vi "2_487.vi"() -> ()   [LabVIEW 2018]
uses:
  <vilib>/Utility/config.llb/Write Key (String).vi
  <vilib>/Utility/config.llb/Read Key (String).vi
  <vilib>/Utility/config.llb/NI_LVConfig.lvlib
panel:
  out "字符串":string
  in  "确定按钮 3":bool
  in  "确定按钮 2":bool
  in  "请输入管理密码":string
  out "CANCEL2":bool
  out "OK2":bool
  out "请输入序列号模板2":string
  out "请输入新产品名称2":string
  in  "?":T1
  in  "工号":string
  in  "工序":string
  in  "取消按钮":bool
  in  "确定按钮":bool
  in  "新建":bool
  out "路径":path
  in  "删除":bool
  in  "产品型号":string(combo)
  # "条形码校验系统配置选择"
  # "新建与删除"
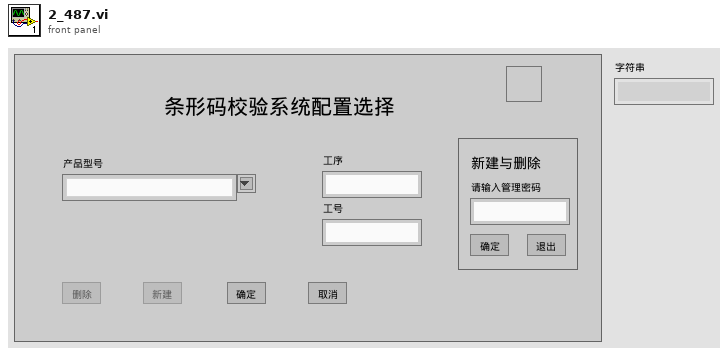
[diagram p1: front panel]
types:
  T1 = cluster{"请输入新产品名称":string, "OK":bool, "CANCEL":bool, "请输入序列号模板":string}
  T2 = enum8{"Enabled", "Disabled", "Disabled and Grayed Out"}
  T3 = typedef "NI_LVConfig.lvlib/Config Data RefNum.ctl" = refnum<k1>
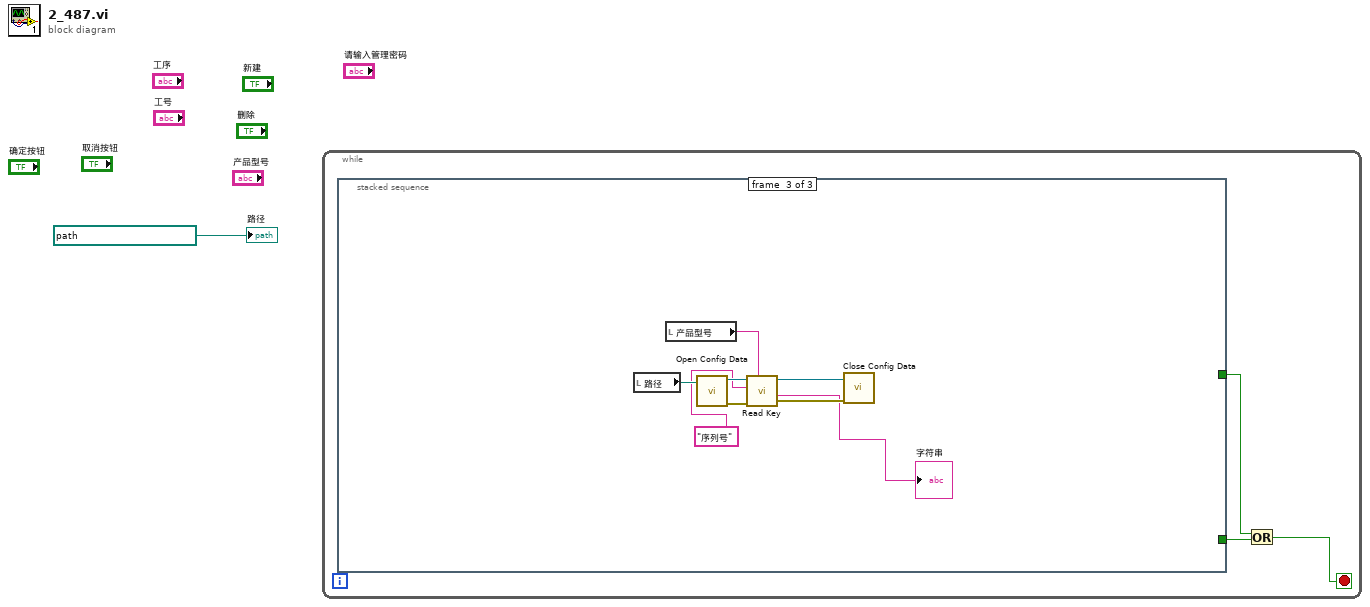
[diagram p0: block diagram]
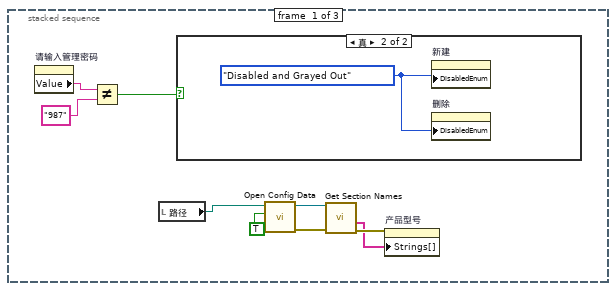
[diagram p2: hidden frame]
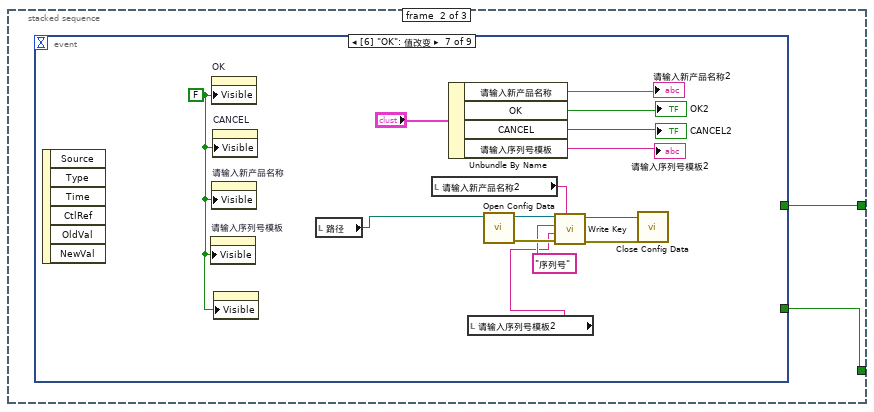
[diagram p4: hidden frame]
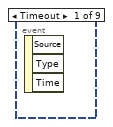
[diagram p5: hidden frame]
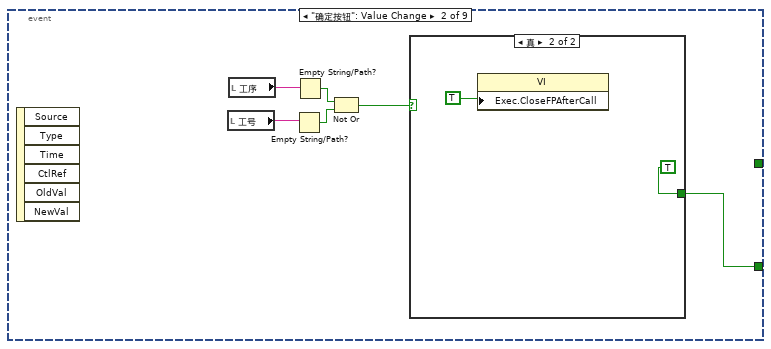
[diagram p6: hidden frame]
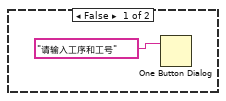
[diagram p7: hidden frame]
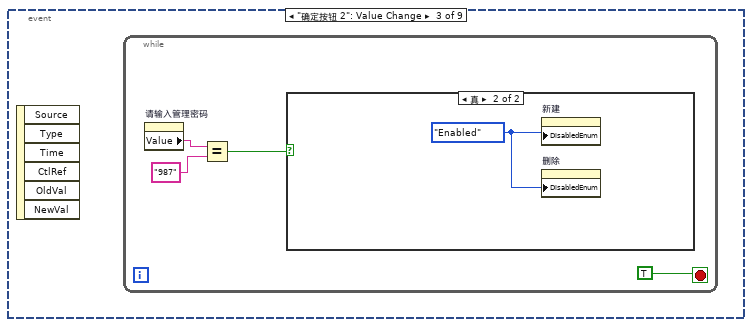
[diagram p8: hidden frame]
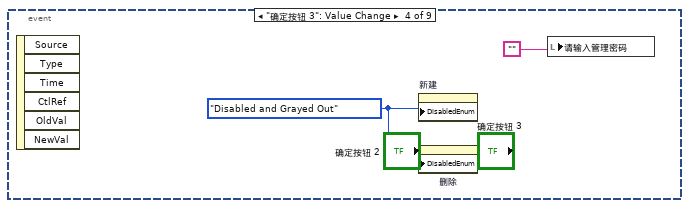
[diagram p10: hidden frame]
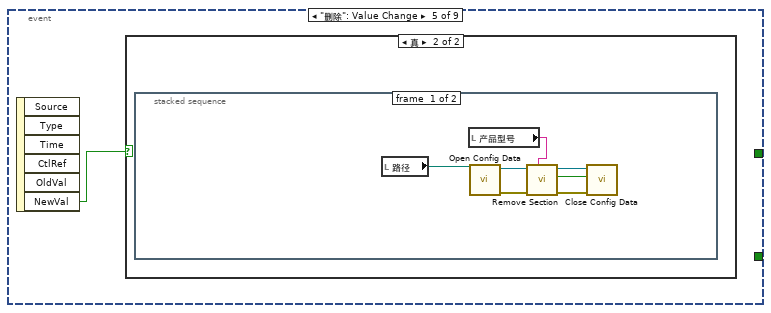
[diagram p11: hidden frame]
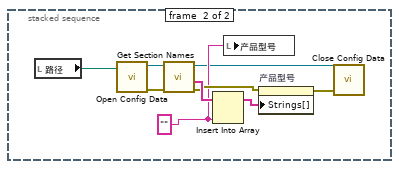
[diagram p13: hidden frame]
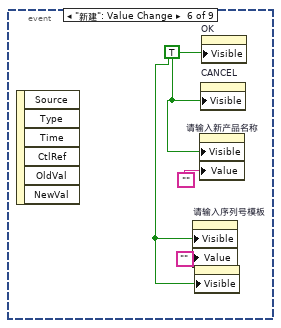
[diagram p14: hidden frame]
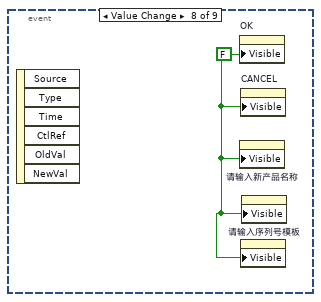
[diagram p15: hidden frame]
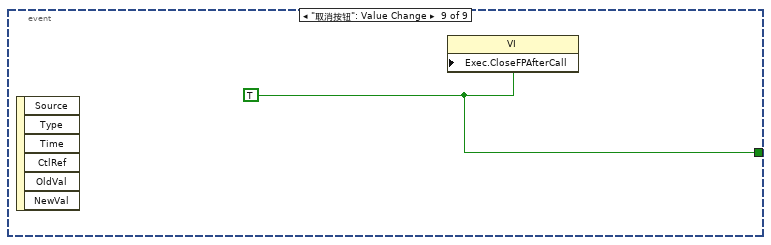
[diagram p16: hidden frame]
diagram:
  n1 = while {
    stop <- w3 stop-if-true
    n2 = stacked-sequence {
      tunnel: [_ w16 _] -> w4
      tunnel: [_ w15 _] -> w2
      frame #0 {
        n3 = property on="请输入管理密码" class="Str"() -> ("Value"=w7:string)  [unwired: 2 in, 2 out]
        n4 = Not Equal?(x=w7, y="987") -> (x != y?=w5:bool)
        n5 = local read "路径"() -> (w8:path)
        n6 = case shown="真" w5 {
          frame False {
          }
          frame True {
            w14 = T2."Disabled and Grayed Out" ("禁用")
            n7 = property on="新建" class="Bool (严格)"("DisabledEnum"=w14) -> ()  [unwired: 2 in, 2 out]
            n8 = property on="删除" class="Bool (严格)"("DisabledEnum"=w14) -> ()  [unwired: 2 in, 2 out]
          }
        }
        n9 = call <vilib>:"Open Config Data.vi"("create file if necessary (T)"=TRUE, "configuration file path"=w8) -> ("error out"=w11:errorcluster, "refnum"=w12:T3)  [unwired: 7 in, 1 out]
        n10 = call <vilib>:"Get Section Names.vi"("error in (no error)"=w11, "refnum"=w12) -> ("error out"=w10:errorcluster, "section names"=w9:string[])  [unwired: 7 in, 1 out]
        n11 = property on="产品型号" class="CmbBox"(error in=w10, "Strings[]"=w9) -> ()  [unwired: 1 in, 2 out]
      }
      frame #1 {
        n12 = event shown="[6] \"OK\": 值改变" {
          selector: _ -> [_ _ _ _ _ _ _ _ _]
          dyn-events: _ -> [_ _ _ _ _ _ _ _ _]
          timeout: _ -> [_ _ _ _ _ _ _ _ _]
          tunnel: [_ w17 _ _ _ _ _ _ _] -> w16
          tunnel: [_ _ _ _ _ _ _ _ w68] -> w15
          event Timeout {
            n13 = event-data() -> ()  [unwired: 1 in, 3 out]
          }
          event "确定按钮": Value Change {
            n14 = event-data() -> ()  [unwired: 1 in, 6 out]
            n15 = local read "工号"() -> (w22:string)
            n16 = local read "工序"() -> (w21:string)
            n17 = Empty String/Path?(string/path=w22) -> (empty?=w19:bool)
            n18 = Empty String/Path?(string/path=w21) -> (empty?=w20:bool)
            n19 = Not Or(1:w19, 2:w20) -> (0:w18:bool)
            n20 = case shown="真" w18 {
              tunnel: [_ TRUE] -> w17
              frame False {
                n21 = One Button Dialog(message="请输入工序和工号") -> ()  [unwired: 1 in, 1 out]
              }
              frame True {
                n22 = property class="VI"("Exec.CloseFPAfterCall"=TRUE) -> ()  [unwired: 2 in, 2 out]
              }
            }
          }
          event "确定按钮 2": Value Change {
            n23 = event-data() -> ()  [unwired: 1 in, 6 out]
            n24 = while {
              stop <- TRUE stop-if-true
              n25 = property on="请输入管理密码" class="Str"() -> ("Value"=w29:string)  [unwired: 2 in, 2 out]
              n26 = Equal?(x=w29, y="987") -> (x = y?=w28:bool)
              n27 = case shown="真" w28 {
                frame False {
                }
                frame True {
                  w30 = T2."Enabled" ("禁用")
                  n28 = property on="新建" class="Bool (严格)"("DisabledEnum"=w30) -> ()  [unwired: 2 in, 2 out]
                  n29 = property on="删除" class="Bool (严格)"("DisabledEnum"=w30) -> ()  [unwired: 2 in, 2 out]
                }
              }
            }
          }
          event "确定按钮 3": Value Change {
            w32 = T2."Disabled and Grayed Out" ("禁用")
            n30 = event-data() -> ()  [unwired: 1 in, 6 out]
            n31 = property on="新建" class="Bool (严格)"("DisabledEnum"=w32) -> ()  [unwired: 2 in, 2 out]
            n32 = property on="删除" class="Bool (严格)"("DisabledEnum"=w32) -> ()  [unwired: 2 in, 2 out]
            n33 = local write "请输入管理密码"("") -> ()
          }
          event "删除": Value Change {
            n34 = event-data() -> ("NewVal"=w33:bool)  [unwired: 1 in, 5 out]
            n35 = case shown="真" w33 {
              frame False {
              }
              frame True {
                n36 = stacked-sequence {
                  frame #0 {
                    n37 = local read "路径"() -> (w34:path)
                    n38 = local read "产品型号"() -> (w40:string)
                    n39 = call <vilib>:"Open Config Data.vi"("configuration file path"=w34) -> ("error out"=w38:errorcluster, "refnum"=w39:T3)  [unwired: 8 in, 1 out]
                    n40 = call <vilib>:"Remove Section.vi"("section"=w40, "error in (no error)"=w38, "refnum"=w39) -> ("error out"=w37:errorcluster, "section exists?"=w36:bool, "refnum out"=w35:T3)  [unwired: 6 in]
                    n41 = call <vilib>:"Close Config Data.vi"("error in (no error)"=w37, "write file if changed (T)"=w36, "refnum"=w35) -> ()  [unwired: 7 in, 2 out]
                  }
                  frame #1 {
                    w44 = ""
                    n42 = local read "路径"() -> (w41:path)
                    n43 = call <vilib>:"Open Config Data.vi"("configuration file path"=w41) -> ("error out"=w49:errorcluster, "refnum"=w48:T3)  [unwired: 8 in, 1 out]
                    n44 = call <vilib>:"Get Section Names.vi"("error in (no error)"=w49, "refnum"=w48) -> ("error out"=w45:errorcluster, "section names"=w47:string[], "refnum out"=w42:T3)  [unwired: 7 in]
                    n45 = Insert Into Array(array=w47, new element=w44) -> (w46:string[])  [unwired: 1 in]
                    n46 = local write "产品型号"(w44) -> ()
                    n47 = property on="产品型号" class="CmbBox"(error in=w45, "Strings[]"=w46) -> (error out=w43:errorcluster)  [unwired: 1 in, 1 out]
                    n48 = call <vilib>:"Close Config Data.vi"("error in (no error)"=w43, "refnum"=w42) -> ()  [unwired: 8 in, 2 out]
                  }
                }
              }
            }
          }
          event "新建": Value Change {
            w51 = TRUE
            n49 = event-data() -> ()  [unwired: 1 in, 6 out]
            n50 = property on="请输入序列号模板" class="Str"("Visible"=w51, "Value"="") -> ()  [unwired: 2 in, 2 out]
            n51 = property class="Clust (严格)"("Visible"=w51) -> ()  [unwired: 2 in, 2 out]
            n52 = property on="请输入新产品名称" class="Str"("Visible"=w51, "Value"="") -> ()  [unwired: 2 in, 2 out]
            n53 = property on="CANCEL" class="Bool (严格)"("Visible"=w51) -> ()  [unwired: 2 in, 2 out]
            n54 = property on="OK" class="Bool (严格)"("Visible"=w51) -> ()  [unwired: 2 in, 2 out]
          }
          event Value Change {
            w58 = FALSE
            n55 = event-data() -> ()  [unwired: 1 in, 6 out]
            n56 = property on="请输入序列号模板" class="Str"("Visible"=w58) -> ()  [unwired: 2 in, 2 out]
            n57 = property on="OK" class="Bool (严格)"("Visible"=w58) -> ()  [unwired: 2 in, 2 out]
            n58 = property on="请输入新产品名称" class="Str"("Visible"=w58) -> ()  [unwired: 2 in, 2 out]
            n59 = property on="CANCEL" class="Bool (严格)"("Visible"=w58) -> ()  [unwired: 2 in, 2 out]
            n60 = property class="Clust (严格)"("Visible"=w58) -> ()  [unwired: 2 in, 2 out]
            n61 = local read "路径"() -> (w66:path)
            n62 = local read "请输入新产品名称2"() -> (w60:string)
            n63 = Unbundle By Name("?") -> ("请输入新产品名称"=→"请输入新产品名称2":string, "OK"=→"OK2":bool, "CANCEL"=→"CANCEL2":bool, "请输入序列号模板"=→"请输入序列号模板2":string)
            n64 = local read "请输入序列号模板2"() -> (w59:string)
            n65 = call <vilib>:"Open Config Data.vi"("configuration file path"=w66) -> ("error out"=w64:errorcluster, "refnum"=w62:T3)  [unwired: 8 in, 1 out]
            n66 = call-poly <vilib>:"Write Key.vi"("section"=w60, "error in (no error)"=w64, "value"=w59, "key"="序列号", "refnum"=w62) -> ("error out"=w65:errorcluster, "refnum out"=w63:T3)  [unwired: 4 in, 1 out]
            n67 = call <vilib>:"Close Config Data.vi"("error in (no error)"=w65, "refnum"=w63) -> ()  [unwired: 8 in, 2 out]
          }
          event Value Change {
            w67 = FALSE
            n68 = event-data() -> ()  [unwired: 1 in, 6 out]
            n69 = property on="OK" class="Bool (严格)"("Visible"=w67) -> ()  [unwired: 2 in, 2 out]
            n70 = property on="请输入新产品名称" class="Str"("Visible"=w67) -> ()  [unwired: 2 in, 2 out]
            n71 = property on="CANCEL" class="Bool (严格)"("Visible"=w67) -> ()  [unwired: 2 in, 2 out]
            n72 = property class="Clust (严格)"("Visible"=w67) -> ()  [unwired: 2 in, 2 out]
            n73 = property on="请输入序列号模板" class="Str"("Visible"=w67) -> ()  [unwired: 2 in, 2 out]
          }
          event "取消按钮": Value Change {
            w68 = TRUE
            n74 = event-data() -> ()  [unwired: 1 in, 6 out]
            n75 = property class="VI"("Exec.CloseFPAfterCall"=w68) -> ()  [unwired: 2 in, 2 out]
          }
        }
      }
      frame #2 {
        n76 = local read "路径"() -> (w71:path)
        n77 = local read "产品型号"() -> (w76:string)
        n78 = call <vilib>:"Open Config Data.vi"("configuration file path"=w71) -> ("error out"=w72:errorcluster, "refnum"=w73:T3)  [unwired: 8 in, 1 out]
        n79 = call-poly <vilib>:"Read Key.vi"("section"=w76, "error in (no error)"=w72, "key"="序列号", "refnum"=w73) -> ("error out"=w75:errorcluster, "value"=→"字符串":string, "refnum out"=w74:T3)  [unwired: 4 in, 1 out]
        n80 = call <vilib>:"Close Config Data.vi"("error in (no error)"=w75, "refnum"=w74) -> ()  [unwired: 8 in, 2 out]
      }
    }
    n81 = Or(x=w2, y=w4) -> (x .or. y?=w3:bool)
  }
  "路径" <- path "D:/扫码防错配置文件.ini" ("基础配置路径")
